vi "QueryLCDC501.vi"(8 "error in (no error)":errorcluster, 11 "VISA resource name":refnum<visa-resource-name>) -> (0 "error out":errorcluster, 1 "LD Voltage":dbl, 2 "LD Current":dbl, 3 "VISA resource name out":refnum<visa-resource-name>, 5 "LD Setting Point":dbl, 7 "Laser status":bool)   [LabVIEW 2021]
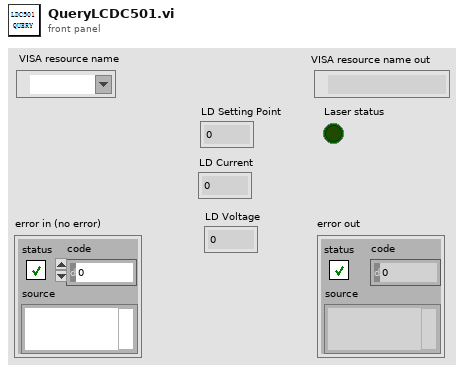
[diagram p1: front panel]
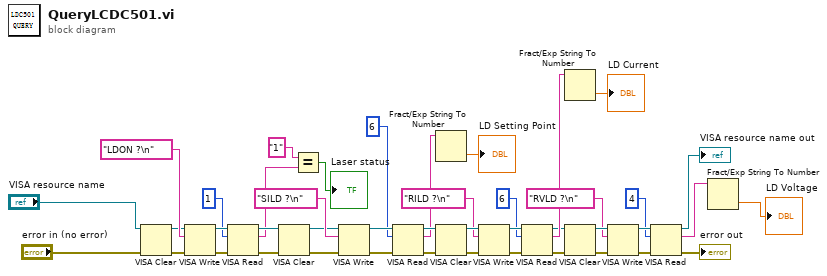
[diagram p0: block diagram]
diagram:
  n1 = VISA Clear(VISA resource name="VISA resource name", error in (no error)="error in (no error)") -> (VISA resource name out=w36:refnum<visa-resource-name>, error out=w37:errorcluster)
  n2 = VISA Write(VISA resource name=w36, write buffer="LDON ?\n", error in (no error)=w37) -> (VISA resource name out=w42:refnum<visa-resource-name>, error out=w41:errorcluster)  [unwired: 1 out]
  n3 = VISA Read(VISA resource name=w42, byte count=u32 1, error in (no error)=w41) -> (VISA resource name out=w30:refnum<visa-resource-name>, read buffer=w14:string, error out=w28:errorcluster)  [unwired: 1 out]
  n4 = VISA Clear(VISA resource name=w30, error in (no error)=w28) -> (VISA resource name out=w29:refnum<visa-resource-name>, error out=w31:errorcluster)
  n5 = Equal?(x="1", y=w14) -> (x = y?=→"Laser status":bool)
  n6 = VISA Write(VISA resource name=w29, write buffer="SILD ?\n", error in (no error)=w31) -> (VISA resource name out=w34:refnum<visa-resource-name>, error out=w35:errorcluster)  [unwired: 1 out]
  n7 = VISA Read(VISA resource name=w34, byte count=u32 6, error in (no error)=w35) -> (VISA resource name out=w23:refnum<visa-resource-name>, read buffer=w19:string, error out=w22:errorcluster)  [unwired: 1 out]
  n8 = Fract/Exp String To Number(string=w19) -> (number=→"LD Setting Point":dbl)  [unwired: 3 in, 1 out]
  n9 = VISA Clear(VISA resource name=w23, error in (no error)=w22) -> (VISA resource name out=w24:refnum<visa-resource-name>, error out=w25:errorcluster)
  n10 = VISA Write(VISA resource name=w24, write buffer="RILD ?\n", error in (no error)=w25) -> (VISA resource name out=w26:refnum<visa-resource-name>, error out=w27:errorcluster)  [unwired: 1 out]
  n11 = VISA Read(VISA resource name=w26, byte count=u32 6, error in (no error)=w27) -> (VISA resource name out=w10:refnum<visa-resource-name>, read buffer=w16:string, error out=w7:errorcluster)  [unwired: 1 out]
  n12 = Fract/Exp String To Number(string=w16) -> (number=→"LD Current":dbl)  [unwired: 3 in, 1 out]
  n13 = VISA Clear(VISA resource name=w10, error in (no error)=w7) -> (VISA resource name out=w9:refnum<visa-resource-name>, error out=w11:errorcluster)
  n14 = VISA Write(VISA resource name=w9, write buffer="RVLD ?\n", error in (no error)=w11) -> (VISA resource name out=w8:refnum<visa-resource-name>, error out=w12:errorcluster)  [unwired: 1 out]
  n15 = VISA Read(VISA resource name=w8, byte count=u32 4, error in (no error)=w12) -> (VISA resource name out=→"VISA resource name out":refnum<visa-resource-name>, read buffer=w3:string, error out=→"error out":errorcluster)  [unwired: 1 out]
  n16 = Fract/Exp String To Number(string=w3) -> (number=→"LD Voltage":dbl)  [unwired: 3 in, 1 out]
